vi "Instrument-Template.doSomethingExample.vi"(8 "error in (no error)":errorcluster, 10 "Data":variant, 11 "Instrument.Framework-Template in":refnum<class "Instrument.Framework-Template.lvclass">) -> (0 "error out":errorcluster, 2 "Data out":variant, 3 "Instrument.Framework-Template out":refnum<class "Instrument.Framework-Template.lvclass">)   [LabVIEW 2019, in "Instrument.Framework-Template.lvclass"]
uses:
  Instrument.Framework-Template.lvclass
  Instrument.Framework-Template.lvclass/Instrument.Framework-Template.ctl
  <userlib>/LevyLab/Instrument Framework/HAL.lvclass
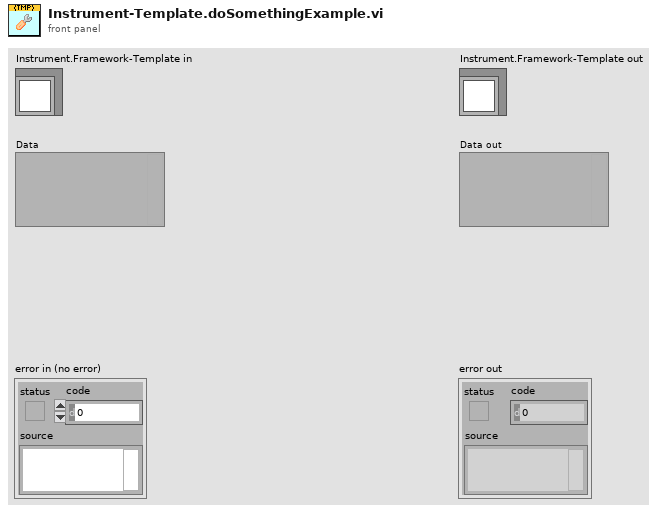
[diagram p1: front panel]
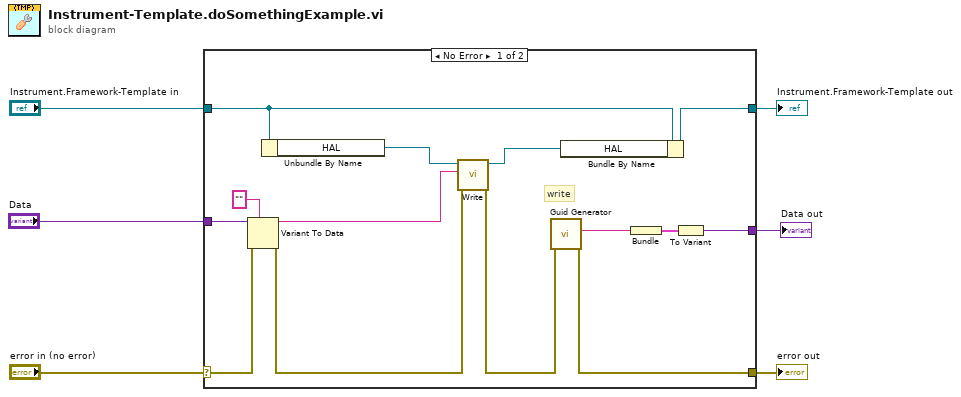
[diagram p0: block diagram]
diagram:
  n1 = case shown="No Error" "error in (no error)" {
    selector: "error in (no error)" -> [w18 w22]
    tunnel: [w16 w22] -> w5
    tunnel: [w7 w21] -> w3
    tunnel: "Instrument.Framework-Template in" -> [w8 w21]
    tunnel: "Data" -> [w20 _]
    tunnel: [w15 _] -> w1
    frame No Error {
      # "write"
      n2 = Variant To Data(error in=w18, type="", Variant=w20) -> (data=w12:string, error out=w11:errorcluster)
      n3 = Unbundle By Name(w8) -> ("HAL"=w10:refnum<class "HAL.lvclass">)
      n4 = call-dynamic "Write.vi"("error in (no error)"=w11, "command"=w12, "HAL in"=w10) -> ("error out"=w13:errorcluster, "HAL out"=w9:refnum<class "HAL.lvclass">)  [unwired: 7 in]
      n5 = call <vilib>:"Guid Generator.vi"("error in (no error)"=w13) -> ("error out"=w16:errorcluster, "GUID"=w17:string)  [unwired: 9 in]
      n6 = Bundle By Name(cluster=w8, "HAL"=w9) -> (w7:refnum<class "Instrument.Framework-Template.lvclass">)
      n7 = Bundle("GUID"=w17) -> (w14:cluster{"GUID":string})  [unwired: 1 in]
      n8 = To Variant(anything=w14) -> (Variant=w15:variant)
    }
    frame Error {
    }
  }
  "error out" <- w5
  "Instrument.Framework-Template out" <- w3
  "Data out" <- w1
